vi "DriveForDistance-C.vi"(11 "Params":string[][](array[string])) -> ()   [LabVIEW 2020]
uses:
  Framework/Robot Global Data.vi
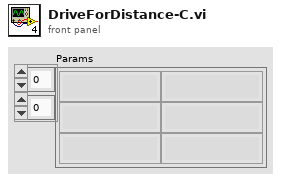
[diagram p1: front panel]
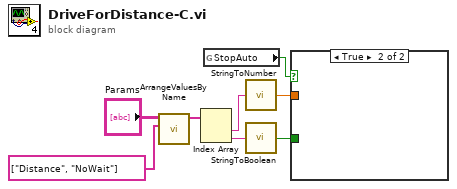
[diagram p0: block diagram]
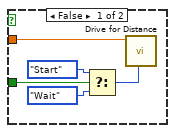
[diagram p2: hidden frame]
diagram:
  n1 = call "ArrangeValuesByName.vi"("Names"=string[] ["Distance", "NoWait"], "Names/Values in"="Params") -> ("Values Out"=w3:string[])  [unwired: 9 in]
  n2 = Index Array(array=w3) -> (element #1=w2:string, element #2=w1:string)  [unwired: 2 in]
  n3 = global read "Robot Global Data.vi" "StopAuto"() -> (w8:bool)
  n4 = call "StringToNumber.vi"("String"=w2) -> ("Output"=w6:dbl)
  n5 = call "StringToBoolean.vi"("String"=w1) -> ("Output"=w7:bool)
  n6 = case shown="True" w8 {
    tunnel: w7 -> [w12 _]
    tunnel: w6 -> [w10 _]
    frame False {
      n7 = Select(t=enum16{"Start", "Wait"}."Start" ("Synchronization"), s=w12, f=enum16{"Start", "Wait"}."Wait" ("Synchronization")) -> (s? t:f=w9:enum16{"Start", "Wait"})
      n8 = call "Drive for Distance.vi"("Synchronication"=w9, "Distance"=w10) -> ()  [unwired: 9 in, 1 out]
    }
    frame True {
    }
  }
